vi "MPC-200 Wrapper for C command.vi"(8 "error in (no error)":errorcluster, 11 "VISA resource name in":refnum<visa-resource-name>) -> (0 "error out":errorcluster, 1 "XYZ Microsteps":u32[](array[numeric]), 2 "Manipulator Number":u8, 3 "VISA resource name out":refnum<visa-resource-name>, 4 "XYZ Microns":dbl[](array[numeric]))   [LabVIEW 2015, in "XYZStage.lvlib"]
uses:
  XYZStage.lvlib
  <vilib>/Utility/error.llb/Error Cluster From Error Code.vi
  <vilib>/ErrorRing/Error Ring.xnode
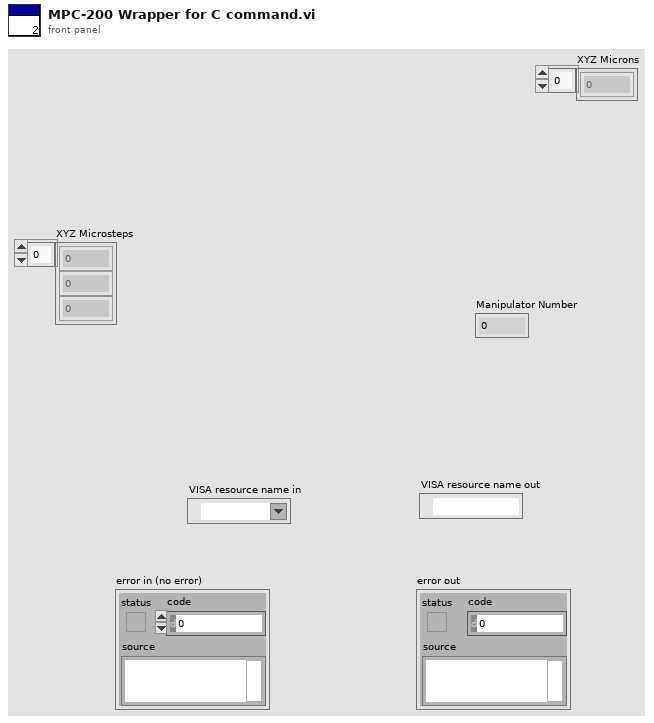
[diagram p1: front panel]
types:
  T1 = enum16{"big-endian, network order", "native, host order", "little-endian"}
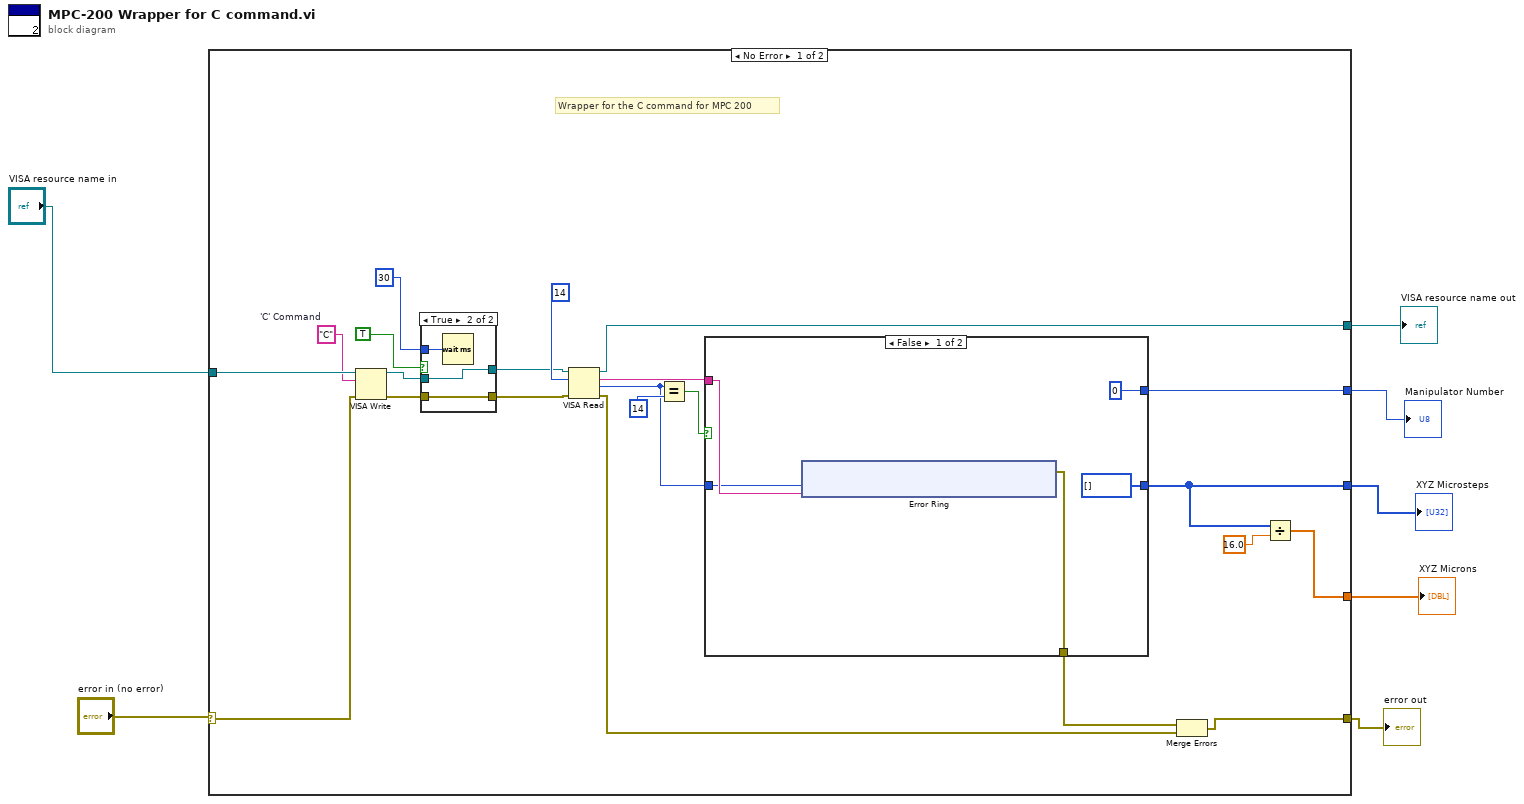
[diagram p0: block diagram]
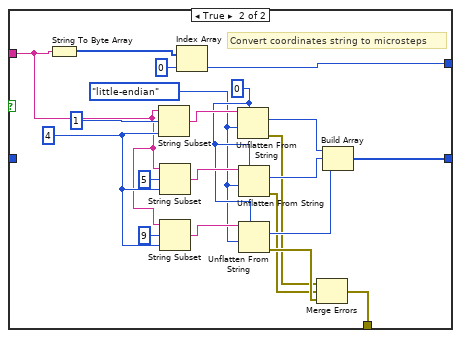
[diagram p3: hidden frame]
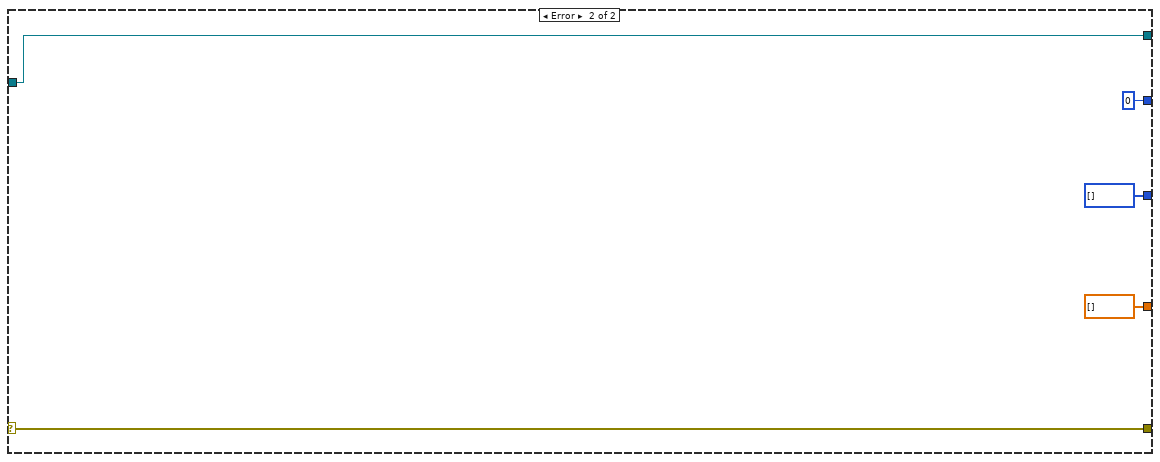
[diagram p4: hidden frame]
diagram:
  n1 = case shown="No Error" "error in (no error)" {
    selector: "error in (no error)" -> [w28 w73]
    tunnel: [w20 w73] -> w6
    tunnel: "VISA resource name in" -> [w29 w72]
    tunnel: [w25 w72] -> w4
    tunnel: [w23 u8 0] -> w3
    tunnel: [w16 u32[] []] -> w2
    tunnel: [w15 dbl[] []] -> w1
    frame No Error {
      w27 = "C"  # 'C' Command
      # "Wrapper for the C command for MPC 200"
      n2 = VISA Write(VISA resource name=w29, write buffer=w27, error in (no error)=w28) -> (VISA resource name out=w11:refnum<visa-resource-name>, error out=w13:errorcluster)  [unwired: 1 out]
      n3 = case shown="True" TRUE {
        tunnel: [w30 w34] -> w14
        tunnel: w13 -> [w30 w34]
        tunnel: [w31 w33] -> w12
        tunnel: w11 -> [w31 w33]
        tunnel: u32 30 ("milliseconds to wait") -> [_ w32]
        frame False {
        }
        frame True {
          n4 = Wait (ms)(milliseconds to wait=w32) -> ()  [unwired: 1 out]
        }
      }
      n5 = VISA Read(VISA resource name=w12, byte count=u32 14, error in (no error)=w14) -> (VISA resource name out=w25:refnum<visa-resource-name>, read buffer=w24:string, return count=w8:u32, error out=w18:errorcluster)
      n6 = Equal?(x=w8, y=u32 14) -> (x = y?=w21:bool)
      n7 = case shown="False" w21 {
        tunnel: w24 -> [w36 w58]
        tunnel: [u8 0 w67] -> w23
        tunnel: [w39 w51] -> w19
        tunnel: [u32[] [] w52] -> w16
        tunnel: w8 -> [w35 _]
        frame False {
          n8 = xnode "Error Ring"("parameter 0"=w35, "parameter 1"=w36) -> ("error out"=w39:errorcluster)
        }
        frame True {
          w56 = T1."little-endian" ("byte order (0:big-endian, network order)")
          w61 = 4 ("length (rest)")
          w57 = u32 0
          # "Convert coordinates string to microsteps"
          n9 = String To Byte Array(string=w58) -> (unsigned byte array=w66:u8[])
          n10 = String Subset(string=w58, offset (0)=1, length (rest)=w61) -> (substring=w64:string)
          n11 = String Subset(string=w58, offset (0)=5, length (rest)=w61) -> (substring=w63:string)
          n12 = String Subset(string=w58, offset (0)=9, length (rest)=w61) -> (substring=w62:string)
          n13 = Index Array(array=w66, index=0) -> (element=w67:u8)
          n14 = Unflatten From String(type=w57, binary string=w64, byte order (0:big-endian, network order)=w56) -> (value=w55:u32, error out=w48:errorcluster)  [unwired: 2 in, 1 out]
          n15 = Unflatten From String(type=w57, binary string=w63, byte order (0:big-endian, network order)=w56) -> (value=w54:u32, error out=w49:errorcluster)  [unwired: 2 in, 1 out]
          n16 = Unflatten From String(type=w57, binary string=w62, byte order (0:big-endian, network order)=w56) -> (value=w53:u32, error out=w50:errorcluster)  [unwired: 2 in, 1 out]
          n17 = Merge Errors(w48, w49, w50) -> (w51:errorcluster)
          n18 = Build Array(w55, w54, w53) -> (w52:u32[])
        }
      }
      n19 = Merge Errors(w19, w18) -> (w20:errorcluster)
      n20 = Divide(x=w16, y=16.0) -> (x/y=w15:dbl[])
    }
    frame Error {
    }
  }
  "VISA resource name out" <- w4
  "error out" <- w6
  "Manipulator Number" <- w3
  "XYZ Microsteps" <- w2
  "XYZ Microns" <- w1
